vi "Кластеры-01-порядок.vi"() -> ()   [LabVIEW 2017]
panel:
  out "Cluster 2":T1
  in  "Cluster":T2
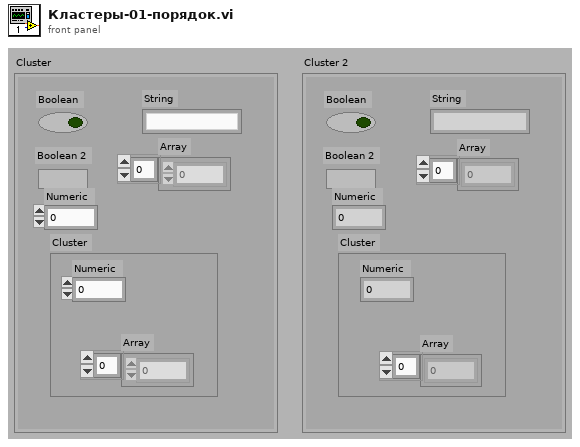
[diagram p1: front panel]
types:
  T1 = cluster{"Array":dbl[], "Cluster":cluster{"Array":u8[], "Numeric":i32}, "Numeric":dbl, "Boolean 2":bool, "String":string, "Boolean":bool}
  T2 = cluster{"Boolean":bool, "Boolean 2":bool, "Numeric":dbl, "String":string, "Array":dbl[], "Cluster":cluster{"Numeric":i32, "Array":u8[]}}
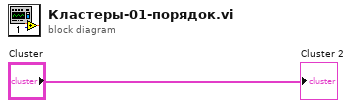
[diagram p0: block diagram]
diagram:
  "Cluster 2" <- "Cluster"
